vi "ODX_Generate Key.vi"(7 "SA2 Operator":T1[](array[typedef]) {"Wert" format="%.0x"}, 11 "Responce with Seed":u8[](array[numeric])=[39, 17] format="%.0x") -> (1 "Key":u8[](array[numeric]) format="%.0x")   [LabVIEW 2014]
uses:
  Typedefs/Diagnose_SA2_Rechnenbefehl.ctl
  Typedefs/Diagnose_SA2_Operation_ENUM.ctl
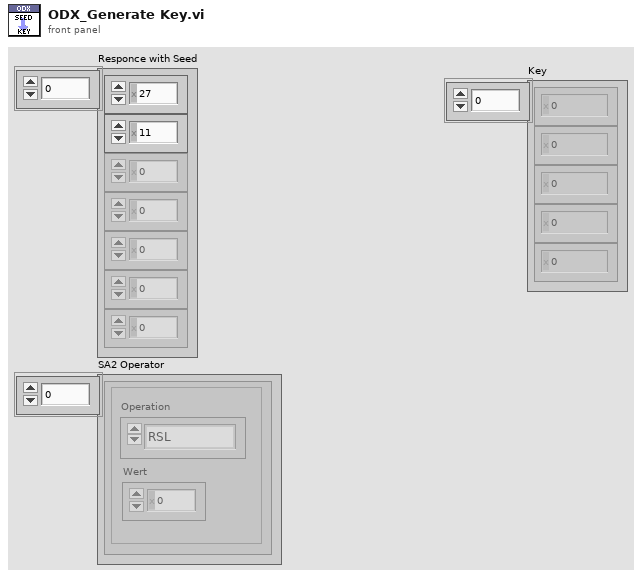
[diagram p1: front panel]
types:
  T1 = typedef "Diagnose_SA2_Rechnenbefehl.ctl" = cluster{"Operation":T2, "Wert":u32}
  T2 = typedef "Diagnose_SA2_Operation_ENUM.ctl" = enum16{"RSL", "RSR", "ADD", "SUB", "EOR", "Durchläufe", "NEXT", "BCC", "BRA", "Fertig"}
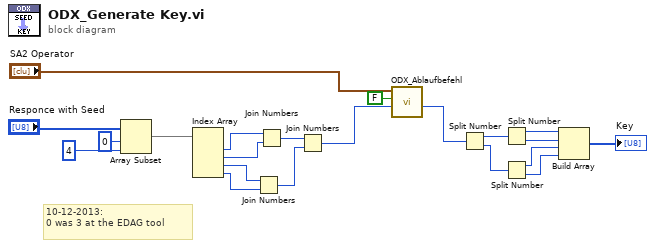
[diagram p0: block diagram]
diagram:
  # "10-12-2013:\n0 was 3 at the EDAG tool"
  n1 = Array Subset(array="Responce with Seed", index=0, length=4) -> (w18:u8[])
  n2 = Index Array(array=w18) -> (element #1=w17:u8, element #2=w16:u8, element #3=w15:u8, element #4=w14:u8)  [unwired: 4 in]
  n3 = Join Numbers(hi=w15, lo=w14) -> ((hi.lo)=w12:u16)
  n4 = Join Numbers(hi=w17, lo=w16) -> ((hi.lo)=w13:u16)
  n5 = Join Numbers(hi=w13, lo=w12) -> ((hi.lo)=w2:u32)
  n6 = call "ODX_Ablaufbefehl.vi"("Operand in"=w2, "Carry in"=FALSE, "SA2 Operator"="SA2 Operator") -> ("Operand out"=w3:u32)  [unwired: 6 in, 2 out]
  n7 = Split Number(x=w3) -> (hi(x)=w11:u16, lo(x)=w10:u16)
  n8 = Split Number(x=w11) -> (hi(x)=w9:u8, lo(x)=w8:u8)
  n9 = Split Number(x=w10) -> (hi(x)=w7:u8, lo(x)=w6:u8)
  n10 = Build Array(w9, w8, w7, w6) -> (→"Key":u8[])
